vi "Logging Configs Directory.vi"() -> (3 "Logging Configs Directory":path)   [LabVIEW 2015, in "Utility.lvlib"]
uses:
  Utility.lvlib
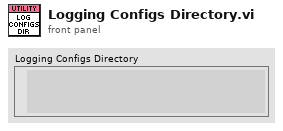
[diagram p1: front panel]
types:
  T1 = typedef "Utility.lvlib/App Paths.ctl" = cluster{"App Ini File":path, "App Data Dir":path, "Config Dir":path, "App Root Dir":path}
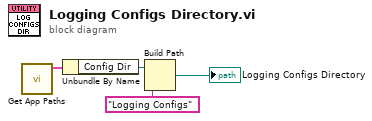
[diagram p0: block diagram]
diagram:
  n1 = call "Get App Paths.vi"() -> ("Paths"=w3:T1)  [unwired: 10 in, 1 out]
  n2 = Unbundle By Name(w3) -> ("Config Dir"=w2:path)
  n3 = Build Path(base path=w2, name or relative path="Logging Configs") -> (appended path=→"Logging Configs Directory":path)
